vi "OSF Format Exp Wiki.vi"(8 "error in":errorcluster, 11 "Proposal Data":T1) -> (0 "error out":errorcluster, 3 "resulting string":string)   [LabVIEW 2020]
uses:
  Calendar/Extract iCalendar String.ctl
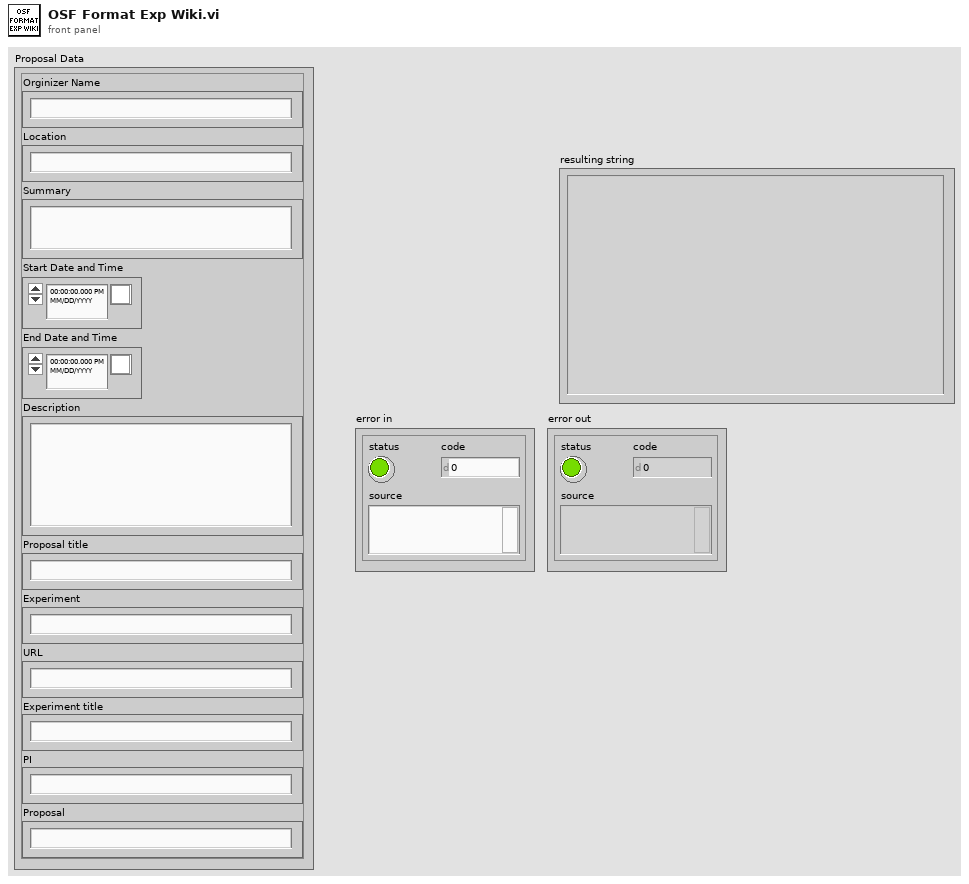
[diagram p1: front panel]
types:
  T1 = typedef "Extract iCalendar String.ctl" = cluster{"Orginizer Name":string, "Location":string, "Summary":string, "Start Date and Time":timestamp, "End Date and Time":timestamp, "Description":string, "Proposal title":string, "Experiment":string, "URL":string, "Experiment title":string, "PI":string, "Proposal":string}
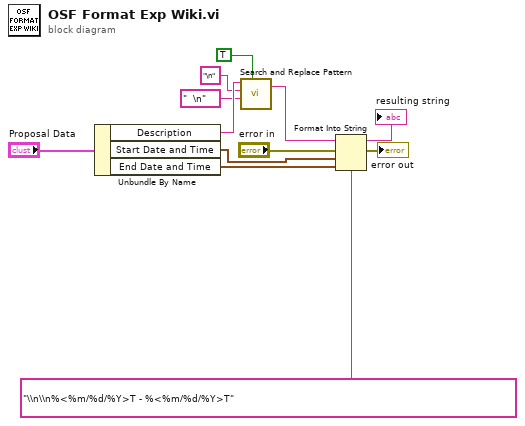
[diagram p0: block diagram]
diagram:
  n1 = Unbundle By Name("Proposal Data") -> ("Description"=w11:string, "Start Date and Time"=w6:timestamp, "End Date and Time"=w5:timestamp)
  n2 = call <vilib>:"Search and Replace Pattern.vi"("string"=w11, "regular expression (\"\")"="\n" ("regular expression (\"\")"), "replace string (\"\")"="  \n" ("regular expression (\"\")"), "replace all? (F)"=TRUE) -> ("result string"=w8:string)  [unwired: 1 in, 1 out]
  n3 = Format Into String(format string="\\n\\n%<%m/%d/%Y>T - %<%m/%d/%Y>T", initial string=w8, error in="error in", w6, w5) -> (resulting string=→"resulting string":string, error out=→"error out":errorcluster)
